vi "Create Cursor Text.vi"(5 "Cursor Text":T3, 6 "Scale":T4, 7 "Cursor Position":T2, 8 "error in (no error)":errorcluster, 10 "Cursor Property":T1, 11 "Cursor Object In":refnum<vi>) -> (0 "error out":errorcluster, 3 "Cursor Object Out":refnum<vi>)   [LabVIEW 2017, in "3D Plot.lvclass"]
uses:
  <vilib>/Math Plots/3D Math Plots/3D Plot/3D Plot/3D Plot.lvclass
  <vilib>/Math Plots/3D Math Plots/3D Plot/3D Plot/Typedef/Cursor Text.ctl
  <vilib>/Math Plots/3D Math Plots/3D Plot/3D Plot/Typedef/Cursor Position.ctl
  <vilib>/picture/3D Picture Control/Object/Create Object (name).vi
  <vilib>/picture/3D Picture Control/NI_3D Picture Control.lvlib
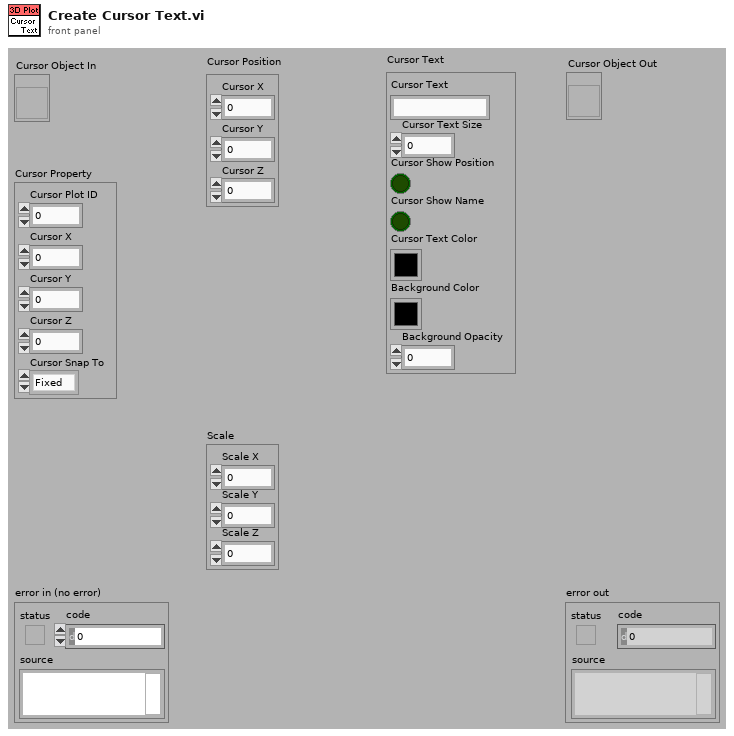
[diagram p1: front panel]
types:
  T1 = typedef "3D Plot.lvclass/Cursor Position.ctl" = cluster{"Cursor Plot ID":i32, "Cursor X":sgl, "Cursor Y":sgl, "Cursor Z":sgl, "Cursor Snap To":enum16{"Fixed", "Nearest Plot", "Snap to Plot"}}
  T2 = cluster{"Cursor X":sgl, "Cursor Y":sgl, "Cursor Z":sgl}
  T3 = typedef "3D Plot.lvclass/Cursor Text.ctl" = cluster{"Cursor Text":string, "Cursor Text Size":u16, "Cursor Show Position":bool, "Cursor Show Name":bool, "Cursor Text Color":u32, "Background Color":u32, "Background Opacity":sgl}
  T4 = cluster{"Scale X":sgl, "Scale Y":sgl, "Scale Z":sgl}
  T5 = enum16{"Normal Bin", "Opaque Bin", "Transparent Bin"}
  T6 = enum16{"Overall", "Per Primitive", "Per Vertex", "Binding Off"}
  T7 = enum16{"Points", "Lines", "Line Strip", "Line Loop", "Triangles", "Triangle Strip", "Triangle Fan", "Quads", "Quad Strip", "Polygon"}
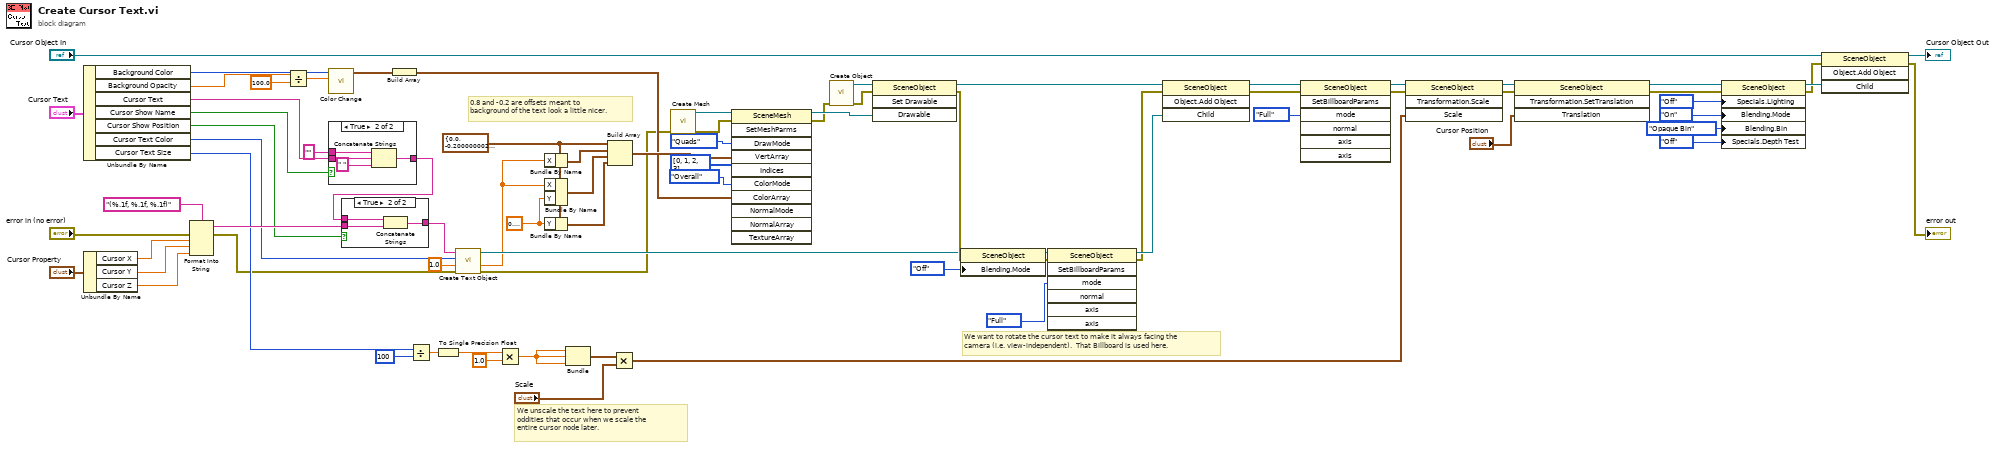
[diagram p0: block diagram]
diagram:
  w67 = sgl 0.8 ("Y")
  w66 = cluster{"X":sgl, "Y":sgl, "Z":sgl} {"X"=0.0, "Y"=-0.2, "Z"=0.0} ("Vect 1")
  # "We want to rotate the cursor text to make it always facing the\ncamera (i.e. view-independent).  That Billboard is used here."
  # "We unscale the text here to prevent oddities that occur when we scale the entire cursor node later."
  # "0.8 and -0.2 are offsets meant to background of the text look a little nicer."
  n1 = Unbundle By Name("Cursor Text") -> ("Background Color"=w69:u32, "Background Opacity"=w22:sgl, "Cursor Text"=w75:string, "Cursor Show Name"=w72:bool, "Cursor Show Position"=w71:bool, "Cursor Text Color"=w18:u32, "Cursor Text Size"=w47:u16)
  n2 = Unbundle By Name("Cursor Property") -> ("Cursor X"=w6:sgl, "Cursor Y"=w5:sgl, "Cursor Z"=w4:sgl)
  n3 = Format Into String(format string="(%.1f, %.1f, %.1f)", error in="error in (no error)", w6, w5, w4) -> (resulting string=w73:string, error out=w26:errorcluster)  [unwired: 1 in]
  n4 = Divide(x=w22, y=100.0) -> (x/y=w21:dbl)
  n5 = call <vilib>:"Color Change.vi"("Alpha"=w21, "Color"=w69) -> ("RGBA"=w70:cluster{"R":sgl, "G":sgl, "B":sgl, "A":sgl})  [unwired: 9 out]
  n6 = case shown="True" w72 {
    tunnel: w75 -> [_ w81]
    tunnel: "" -> [w78 w82]
    tunnel: [w78 w79] -> w77
    frame False {
    }
    frame True {
      n7 = Concatenate Strings(w82, w81, " " ("string")) -> (w79:string)
    }
  }
  n8 = case shown="True" w71 {
    tunnel: w77 -> [w83 w86]
    tunnel: w73 -> [_ w85]
    tunnel: [w83 w84] -> w27
    frame False {
    }
    frame True {
      n9 = Concatenate Strings(w86, w85) -> (w84:string)
    }
  }
  n10 = Build Array(w70) -> (w57:cluster{"R":sgl, "G":sgl, "B":sgl, "A":sgl}[])
  n11 = Divide(x=w47, y=100) -> (x/y=w49:dbl)
  n12 = To Single Precision Float(number=w49) -> (single precision float=w7:sgl)
  n13 = call <vilib>:"Create Text Object.vi"("error in (no error)"=w26, "Alpha"=sgl 1.0, "Color Box"=w18, "Value String"=w27) -> ("error out"=w23:errorcluster, "Numeric"=w24:sgl, "Scene:New Object"=w25:refnum<vi>)  [unwired: 5 out]
  n14 = Multiply(x=w7, y=sgl 1.0 ("Length")) -> (x*y=w50:sgl)
  n15 = Bundle By Name(cluster=w66, "X"=w24) -> (w68:cluster{"X":sgl, "Y":sgl, "Z":sgl})
  n16 = Bundle By Name(cluster=w66, "X"=w24, "Y"=w67) -> (w65:cluster{"X":sgl, "Y":sgl, "Z":sgl})
  n17 = Bundle By Name(cluster=w66, "Y"=w67) -> (w64:cluster{"X":sgl, "Y":sgl, "Z":sgl})
  n18 = Bundle(w50, w50, w50) -> (w51:cluster{sgl, sgl, sgl})  [unwired: 1 out]
  n19 = Build Array(w66, w68, w65, w64) -> (w61:cluster{"X":sgl, "Y":sgl, "Z":sgl}[])
  n20 = Multiply(x=w51, y="Scale") -> (x*y=w42:cluster{sgl, sgl, sgl})
  n21 = call <vilib>:"Create Mesh.vi"("error in (no error)"=w23) -> ("error out"=w62:errorcluster, "New Mesh Refnum"=w63:refnum<vi>)  [unwired: 9 out]
  n22 = invoke class="SceneMesh" method="SetMeshParms"(reference=w63, error in=w62, "DrawMode"=T7."Quads" ("Draw Mode"), "VertArray"=w61, "Indices"=u32[] [0, 1, 2, 3], "ColorMode"=T6."Overall" ("Color Binding Mode"), "ColorArray"=w57) -> (reference out=w55:refnum<vi>, error out=w35:errorcluster)  [unwired: 4 in, 9 out]
  n23 = call-poly <vilib>:"Create Object.vi"("error in (no error)"=w35) -> ("error out"=w34:errorcluster, "Scene:New Object"=w56:refnum<vi>)  [unwired: 9 in]
  n24 = invoke class="SceneObject" method="Set Drawable"(reference=w56, error in=w34, "Drawable"=w55) -> (reference out=w54:refnum<vi>, error out=w33:errorcluster)  [unwired: 1 in, 2 out]
  n25 = property class="SceneObject"(reference=w25, error in=w33, "Blending.Mode"=enum16{"Inherit Value", "Off", "On"}."Off" ("Blending:Mode")) -> (reference out=w11:refnum<vi>, error out=w9:errorcluster)
  n26 = invoke class="SceneObject" method="SetBillboardParams"(reference=w11, error in=w9, "mode"=enum16{"No Billboarding", "Axial", "Full"}."Full") -> (reference out=w10:refnum<vi>, error out=w8:errorcluster)  [unwired: 4 in, 5 out]
  n27 = invoke class="SceneObject" method="Object.Add Object"(reference=w54, error in=w8, "Child"=w10) -> (reference out=w16:refnum<vi>, error out=w15:errorcluster)  [unwired: 1 in, 2 out]
  n28 = invoke class="SceneObject" method="SetBillboardParams"(reference=w16, error in=w15, "mode"=enum16{"No Billboarding", "Axial", "Full"}."Full") -> (reference out=w14:refnum<vi>, error out=w13:errorcluster)  [unwired: 4 in, 5 out]
  n29 = invoke class="SceneObject" method="Transformation.Scale"(reference=w14, error in=w13, "Scale"=w42) -> (reference out=w43:refnum<vi>, error out=w32:errorcluster)  [unwired: 1 in, 2 out]
  n30 = invoke class="SceneObject" method="Transformation.SetTranslation"(reference=w43, error in=w32, "Translation"="Cursor Position") -> (reference out=w40:refnum<vi>, error out=w31:errorcluster)  [unwired: 1 in, 2 out]
  n31 = property class="SceneObject"(reference=w40, error in=w31, "Specials.Lighting"=enum16{"Inherit Value", "Off", "On"}."Off" ("Specials:Lighting"), "Blending.Mode"=enum16{"Inherit Value", "Off", "On"}."On" ("Blending:Mode"), "Blending.Bin"=T5."Opaque Bin" ("Blending:Bin"), "Specials.Depth Test"=enum16{"Inherit Value", "Off", "On"}."Off" ("Specials:Depth Test")) -> (reference out=w39:refnum<vi>, error out=w30:errorcluster)
  n32 = invoke class="SceneObject" method="Object.Add Object"(reference="Cursor Object In", error in=w30, "Child"=w39) -> (reference out=→"Cursor Object Out":refnum<vi>, error out=→"error out":errorcluster)  [unwired: 1 in, 2 out]
